vi "comm get ring.vi"(8 "error in (no error)":errorcluster, 11 "Comm Handle":u64) -> (0 "error out":errorcluster, 2 "RING":bool, 3 "dup Comm Handle":u64)   [LabVIEW 2009, in "lvserial.lvlib"]
doc: "Retrieves modem control-register values."
uses:
  lvserial.lvlib
  x64/Release/lvserial.dll
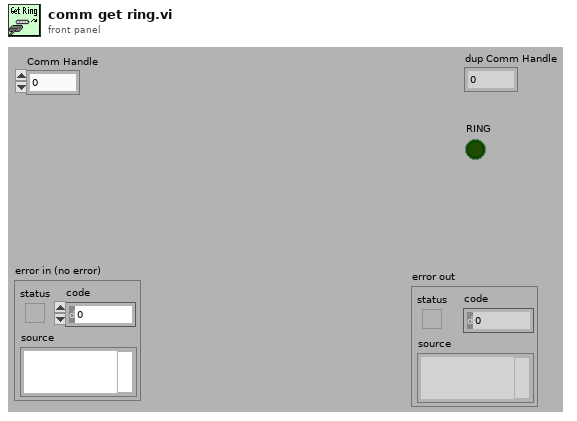
[diagram p1: front panel]
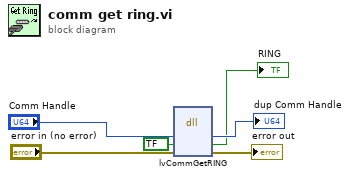
[diagram p0: block diagram]
diagram:
  n1 = dll-call lib="C:/Users/Admin/Desktop/lvserial_source_1-2-13/x64/Release/lvserial.dll" fn="lvCommGetRING"("hComm"="Comm Handle", "pfRING"=bool ? ("CTS"), "error"="error in (no error)") -> ("hComm"=→"dup Comm Handle":u64, "pfRING"=→"RING":bool, "error"=→"error out":errorcluster)  [unwired: 3 in, 3 out]
